vi "Crossover.vi"(8 "error in (no error)":errorcluster, 11 "TSP Class in":refnum<class "TSP Class.lvclass">) -> (0 "error out":errorcluster, 3 "TSP Class out":refnum<class "TSP Class.lvclass">)   [LabVIEW 2015, in "TSP Library.lvlib" / "TSP Class.lvclass"]
uses:
  TSP Class.lvclass
  TSP Class.lvclass/TSP Class.ctl
  TSP Library.lvlib
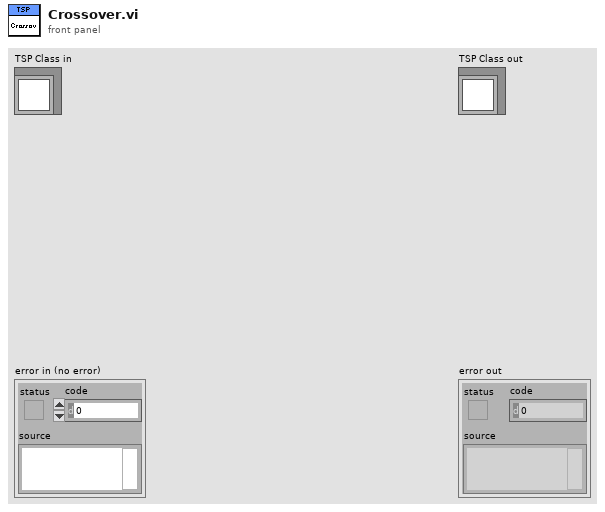
[diagram p1: front panel]
types:
  T1 = typedef "TSP Library.lvlib/Path.ctl" = cluster{"Distance":dbl, "Tour":i32[]}
  T2 = typedef "TSP Library.lvlib/Crossover.ctl" = enum16{"empty", "Pair v1", "Pair v2", "Pair v3", "Roulette v1", "Roulette v2", "Roulette v3"}
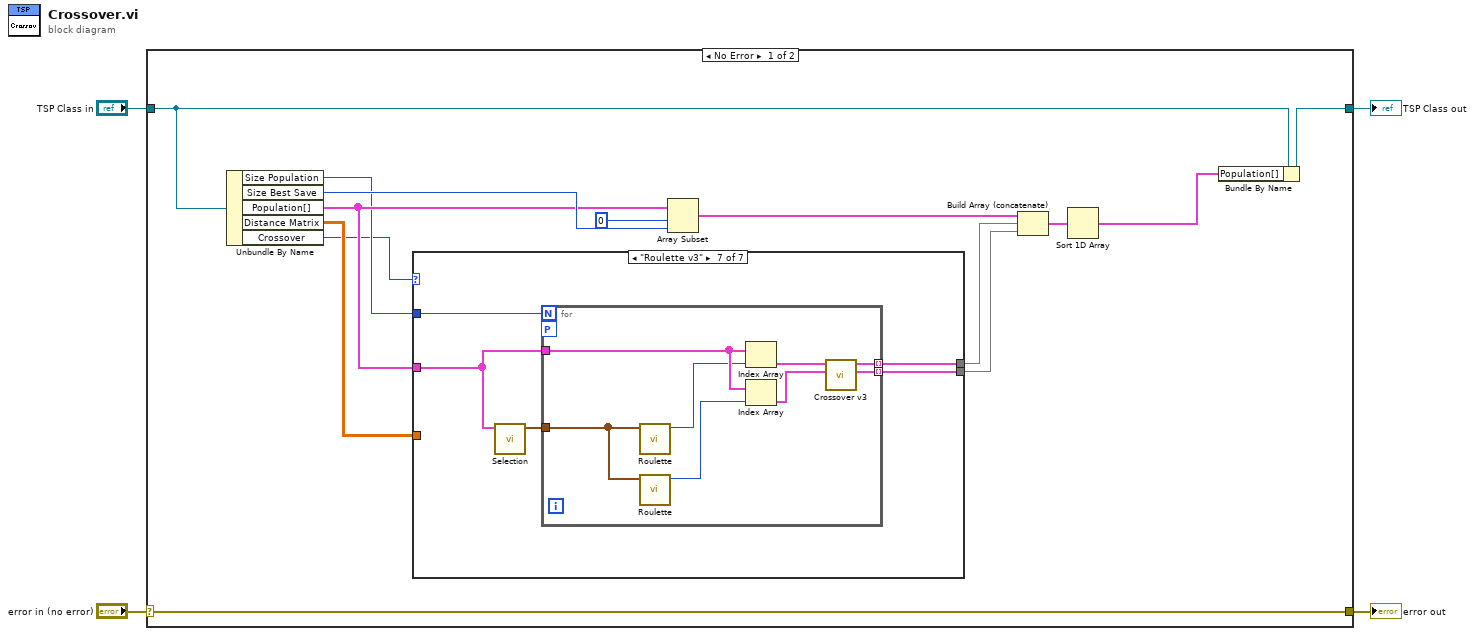
[diagram p0: block diagram]
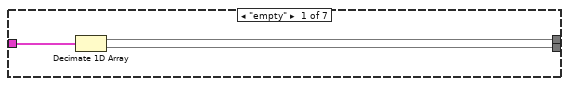
[diagram p2: hidden frame]
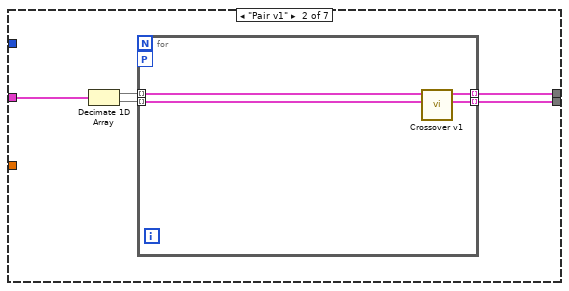
[diagram p3: hidden frame]
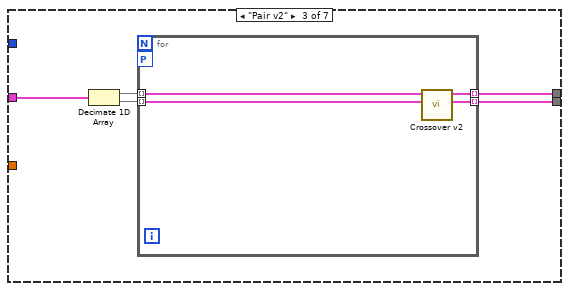
[diagram p4: hidden frame]
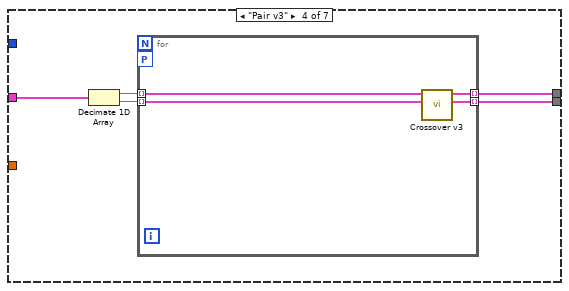
[diagram p5: hidden frame]
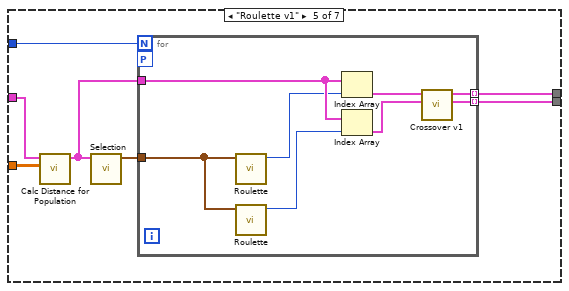
[diagram p6: hidden frame]
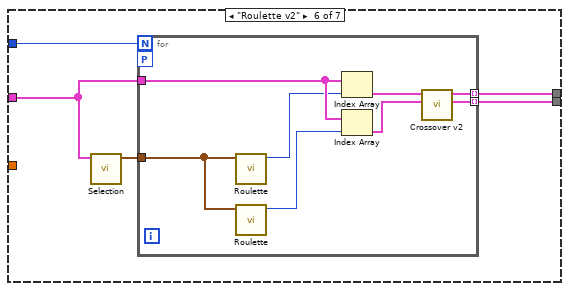
[diagram p7: hidden frame]
diagram:
  n1 = case shown="No Error" "error in (no error)" {
    selector: "error in (no error)" -> [w18 w91]
    tunnel: [w18 w91] -> w1
    tunnel: [w11 w90] -> w3
    tunnel: "TSP Class in" -> [w17 w90]
    frame No Error {
      n2 = Unbundle By Name(w17) -> ("Size Population"=w7:u16, "Size Best Save"=w15:u16, "Population[]"=w9:T1[], "Distance Matrix"=w8:dbl[][], "Crossover"=w6:T2)
      n3 = case shown="\"Roulette v3\"" w6 {
        tunnel: [w20 w26 w35 w44 w55 w68 w81] -> w13
        tunnel: [w19 w25 w34 w43 w54 w67 w80] -> w10
        tunnel: w9 -> [w21 w24 w33 w42 w51 w64 w77]
        tunnel: w8 -> [_ _ _ _ w52 _ _]
        tunnel: w7 -> [_ _ _ _ w49 w65 w78]
        frame "empty" {
          n4 = Decimate 1D Array(w21) -> (w20:T1[], w19:T1[])
        }
        frame "Pair v1" {
          n5 = Decimate 1D Array(w24) -> (w23:T1[], w22:T1[])
          n6 = for {
            tunnel: [w30] -> w26 mode=indexing
            workers-P: _ -> [_]
            tunnel: [w29] -> w25 mode=indexing
            tunnel: w23 -> [w27] mode=indexing
            tunnel: w22 -> [w28] mode=indexing
            n7 = call "Crossover v1.vi"("Path In 2"=w28, "Path In 1"=w27) -> ("Path Out 2"=w29:T1, "Path Out 1"=w30:T1)  [unwired: 8 in]
          }
        }
        frame "Pair v2" {
          n8 = Decimate 1D Array(w33) -> (w32:T1[], w31:T1[])
          n9 = for {
            tunnel: [w39] -> w35 mode=indexing
            workers-P: _ -> [_]
            tunnel: [w38] -> w34 mode=indexing
            tunnel: w32 -> [w36] mode=indexing
            tunnel: w31 -> [w37] mode=indexing
            n10 = call "Crossover v2.vi"("Path In 2"=w37, "Path In 1"=w36) -> ("Path Out 2"=w38:T1, "Path Out 1"=w39:T1)  [unwired: 8 in]
          }
        }
        frame "Pair v3" {
          n11 = Decimate 1D Array(w42) -> (w41:T1[], w40:T1[])
          n12 = for {
            tunnel: [w48] -> w44 mode=indexing
            workers-P: _ -> [_]
            tunnel: [w47] -> w43 mode=indexing
            tunnel: w41 -> [w45] mode=indexing
            tunnel: w40 -> [w46] mode=indexing
            n13 = call "Crossover v3.vi"("Path In 2"=w46, "Path In 1"=w45) -> ("Path Out 2"=w47:T1, "Path Out 1"=w48:T1)  [unwired: 8 in]
          }
        }
        frame "Roulette v1" {
          n14 = call "Calc Distance for Population.vi"("Distance Matrix"=w52, "Population[] In"=w51) -> ("Population[] Out"=w50:T1[])  [unwired: 9 in]
          n15 = call "Selection.vi"("Population[]"=w50) -> ("Range"=w53:cluster{dbl, dbl}[])  [unwired: 10 in]
          n16 = for {
            N: w49 -> [_]
            tunnel: [w63] -> w55 mode=indexing
            workers-P: _ -> [_]
            tunnel: [w62] -> w54 mode=indexing
            tunnel: w53 -> [w58]
            tunnel: w50 -> [w60]
            n17 = call "Roulette.vi"("Range"=w58) -> ("Index"=w57:i32)  [unwired: 10 in]
            n18 = call "Roulette.vi"("Range"=w58) -> ("Index"=w56:i32)  [unwired: 10 in]
            n19 = Index Array(array=w60, index=w57) -> (element=w61:T1)
            n20 = Index Array(array=w60, index=w56) -> (element=w59:T1)
            n21 = call "Crossover v1.vi"("Path In 2"=w59, "Path In 1"=w61) -> ("Path Out 2"=w62:T1, "Path Out 1"=w63:T1)  [unwired: 8 in]
          }
        }
        frame "Roulette v2" {
          n22 = call "Selection.vi"("Population[]"=w64) -> ("Range"=w66:cluster{dbl, dbl}[])  [unwired: 10 in]
          n23 = for {
            N: w65 -> [_]
            tunnel: [w76] -> w68 mode=indexing
            workers-P: _ -> [_]
            tunnel: [w75] -> w67 mode=indexing
            tunnel: w66 -> [w71]
            tunnel: w64 -> [w73]
            n24 = call "Roulette.vi"("Range"=w71) -> ("Index"=w70:i32)  [unwired: 10 in]
            n25 = call "Roulette.vi"("Range"=w71) -> ("Index"=w69:i32)  [unwired: 10 in]
            n26 = Index Array(array=w73, index=w70) -> (element=w74:T1)
            n27 = Index Array(array=w73, index=w69) -> (element=w72:T1)
            n28 = call "Crossover v2.vi"("Path In 2"=w72, "Path In 1"=w74) -> ("Path Out 2"=w75:T1, "Path Out 1"=w76:T1)  [unwired: 8 in]
          }
        }
        frame "Roulette v3" {
          n29 = call "Selection.vi"("Population[]"=w77) -> ("Range"=w79:cluster{dbl, dbl}[])  [unwired: 10 in]
          n30 = for {
            N: w78 -> [_]
            tunnel: [w89] -> w81 mode=indexing
            workers-P: _ -> [_]
            tunnel: [w88] -> w80 mode=indexing
            tunnel: w79 -> [w84]
            tunnel: w77 -> [w86]
            n31 = call "Roulette.vi"("Range"=w84) -> ("Index"=w83:i32)  [unwired: 10 in]
            n32 = call "Roulette.vi"("Range"=w84) -> ("Index"=w82:i32)  [unwired: 10 in]
            n33 = Index Array(array=w86, index=w83) -> (element=w87:T1)
            n34 = Index Array(array=w86, index=w82) -> (element=w85:T1)
            n35 = call "Crossover v3.vi"("Path In 2"=w85, "Path In 1"=w87) -> ("Path Out 2"=w88:T1, "Path Out 1"=w89:T1)  [unwired: 8 in]
          }
        }
      }
      n36 = Array Subset(array=w9, index=0, length=w15) -> (w14:T1[])
      n37 = Build Array (concatenate)(w14, w13, w10) -> (w12:T1[])
      n38 = Sort 1D Array(array=w12) -> (sorted array=w5:T1[])
      n39 = Bundle By Name(cluster=w17, "Population[]"=w5) -> (w11:refnum<class "TSP Class.lvclass">)
    }
    frame Error {
    }
  }
  "error out" <- w1
  "TSP Class out" <- w3
